vi "Zero-Order Hold PtByPt.vi"(1 "initialize":bool, 2 "hold time in cycles":i32, 3 "input data point":dbl format="%0.2f") -> (0 "output data point":dbl format="%0.2f")   [LabVIEW 2017, in "NI_PtbyPt.lvlib"]
doc: "Holds <B>input data point</B> for the <B>hold time in cycles</B> that you define. In other words, <B>output data point</B> is a delayed instance of <B>input data point</B>."
uses:
  <vilib>/ptbypt/NI_PtbyPt.lvlib
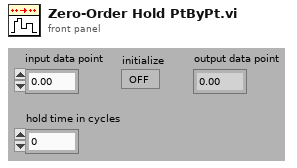
[diagram p1: front panel]
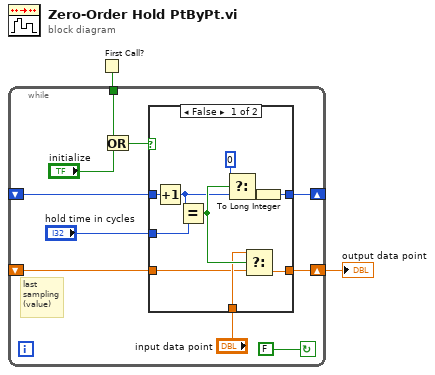
[diagram p0: block diagram]
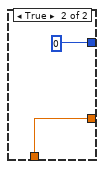
[diagram p2: hidden frame]
diagram:
  n1 = First Call?() -> (First Call?: T/F=w1:bool)
  n2 = while {
    tunnel: w1 -> [w4]
    shift-left: _ -> [w10]
    shift-right: [w11] -> _
    shift-left: _ -> [w9]
    shift-right: [w12] -> w2
    stop <- FALSE continue-if-true
    # "last\nsampling\n(value)"
    n3 = Or(x=w4, y="initialize") -> (x .or. y?=w5:bool)
    n4 = case shown="False" w5 {
      tunnel: [w13 0] -> w11
      tunnel: [w14 w23] -> w12
      tunnel: w10 -> [w22 _]
      tunnel: w9 -> [w15 _]
      tunnel: "input data point" -> [w16 w23]
      tunnel: "hold time in cycles" -> [w21 _]
      frame False {
        n5 = Increment(x=w22) -> (x+1=w19:i32)
        n6 = Equal?(x=w19, y=w21) -> (x = y?=w20:bool)
        n7 = Select(t=0, s=w20, f=w19) -> (s? t:f=w17:i32)
        n8 = Select(t=w16, s=w20, f=w15) -> (s? t:f=w14:dbl)
        n9 = To Long Integer(number=w17) -> (32bit integer=w13:i32)
      }
      frame True {
      }
    }
  }
  "output data point" <- w2
